vi "init.vi"(7 "Prepend Result Name":bool, 8 "error in (no error)":errorcluster, 9 "SA Pin":string, 10 "Measurement Times (s)":dbl[](array[numeric]), 11 "Measurement Name":string) -> (0 "error out":errorcluster, 3 "Skyworks_PA_Modeswitch_out":refnum<class "Skyworks_PA_Modeswitch.lvclass">)   [LabVIEW 2016, in "SeqAuto Evaluations.lvlib" / "Skyworks_PA_Modeswitch.lvclass"]
uses:
  Skyworks_PA_Modeswitch.lvclass
  C:/Sequence Automation/Plugins/SeqAuto IEvaluation.lvlibp/SeqAuto IEvaluation.lvclass
  Skyworks_PA_Modeswitch.lvclass/Skyworks_PA_Modeswitch.ctl
  Plugins/SeqAuto IEvaluation.lvlibp/Write Measurement Name.vi
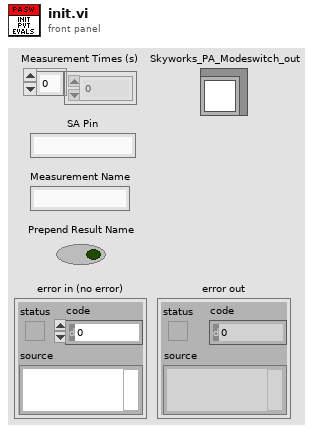
[diagram p1: front panel]
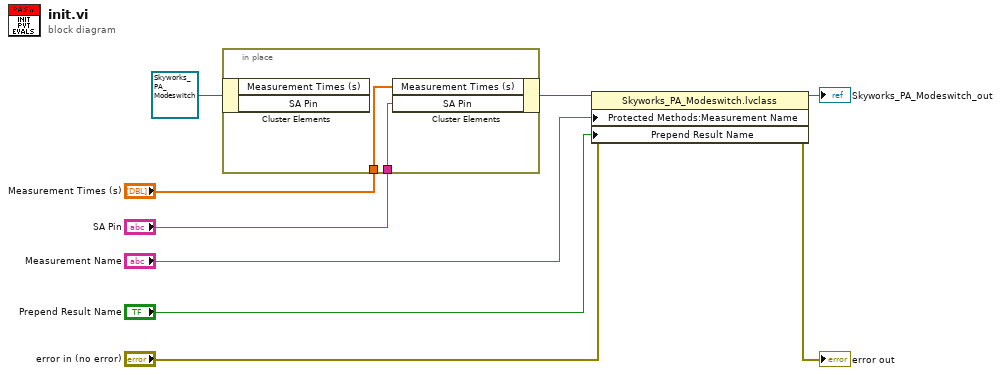
[diagram p0: block diagram]
diagram:
  n1 = in-place {
    in-place-border: "Measurement Times (s)" -> [w11]
    in-place-border: "SA Pin" -> [w10]
    n2 = in-place-cluster #1(refnum<class "Skyworks_PA_Modeswitch.lvclass"> refnum ("Skyworks_2G_PVT in")) -> ()  [unwired: 2 out]
    n3 = in-place-cluster #1("Measurement Times (s)"=w11, "SA Pin"=w10) -> (w5:refnum<class "Skyworks_PA_Modeswitch.lvclass">)
  }
  n4 = property class="Skyworks_PA_Modeswitch.lvclass"(reference=w5, error in="error in (no error)", "Protected Methods:Measurement Name"="Measurement Name", "Prepend Result Name"="Prepend Result Name") -> (reference out=→"Skyworks_PA_Modeswitch_out":refnum<class "Skyworks_PA_Modeswitch.lvclass">, error out=→"error out":errorcluster)
